vi "FPGA_main.vi"   [LabVIEW 2015]
uses:
  CONTROLS/Q_main_element.ctl
  CONTROLS/Q_FPGA_element.ctl
  GLOBAL/Global_FPGA.vi
  GLOBAL/Global_ABORT.vi
  GLOBAL/Global_MAIN.vi
  <vilib>/FPGAPlugInAG/Dynamic/niLvFpga_Reset_Dynamic.vi
  <vilib>/FPGAPlugInAG/Dynamic/niLvFpga_Close_Dynamic.vi
  <vilib>/FPGAPlugInAG/PCIe-7841R/niLvFpga_Open_PCIe-7841R.vi
  <vilib>/rvi/interface/common/dynamic/niFpgaDynamicAddResources.vi
  <vilib>/Utility/error.llb/Error Cluster From Error Code.vi
  <vilib>/rvi/errors/niLvFpgaAdjustHostInterfaceError.vi
  <vilib>/FPGAPlugInAG/Dynamic/niLvFpga_Run_Dynamic.vi
  <vilib>/FPGAPlugInAG/Dynamic/niLvFpga_Abort_Dynamic.vi
  <vilib>/rvi/interface/nirviMethod/nirviMethod.xnode
  <vilib>/rvi/interface/nirviCloseFPGA/nirviCloseFPGA.xnode
  <vilib>/rvi/interface/nirviOpenFPGA/nirviOpenFPGA.xnode
  FPGA/FPGA Bitfiles/FPGAv0_FPGATarget_FPGAlasercontrol_rVrWu38G2Ac.lvbitx
  <vilib>/rvi/interface/nirviReadWriteControl/nirviReadWriteControl.xnode
  FPGA/FPGA Bitfiles/FPGAv0_FPGATarget_FPGAmeasureQPDsi_91djMVJ3FxY.lvbitx
  FPGA/FPGA Bitfiles/FPGAv0_FPGATarget_FPGAtriggercamer_8mvrEZH3eNo.lvbitx
  FPGA/FPGA Bitfiles/FPGAv0_FPGATarget_FPGAmerFISHtrigg_IvsmFeOu1pU.lvbitx
  NiFpgaLv.dll
  <vilib>/rvi/interface/Simulation/niFpgaSimulationCallBeginRW.vi
types:
  T1 = cluster{"N laser lines":i32, "N Z positions":i32, "Laser lines":i32[], "Laser power":sgl[]}
  T2 = typedef "Q_FPGA_element.ctl" = cluster{"variant":variant, "Instruction":enum16{"FPGA_idle", "FPGA_initialize", "FPGA_error", "FPGA_security_stop", "FPGA_laser", "FPGA_start_stop_measure_QPD", "FPGA_measure_QPD", "FPGA_measure_QPD_noise", "FPGA_stop_measure_QPD", "FPGA_init_autofocus", "FPGA_init_single_scan", "FPGA_stop_single_scan", "FPGA_init_merFISH", "FPGA_measure_QPD_merFISH", "FPGA_init_scan_merFISH", "FPGA_scan_merFISH", "FPGA_close_merFISH", "FPGA_stop"}}
  T3 = typedef "Q_main_element.ctl" = cluster{"variant":variant, "Instruction":enum16{"Main_idle", "Main_initialize", "Main_initialize_TDMS", "Main_initialize_Queue", "Main_error", "Main_DAQ_initialization_results", "Main_ASI_initialization_results", "Main_Piezo_initialization_results", "Main_Valve_initialization_results", "Main_Pump_initialization_results", "Main_CAMERA_initialization_results", "Main_FPGA_initialization_results", "Main_DAQ_error", "Main_ASI_error", "Main_Piezo_error", "Main_CAMERA_error", "Main_Valve_error", "Main_Pump_error", "Main_FPGA_error", "Main_start_acquiring", "Main_not_acquiring", "Main_acquiring", "Main_stop_acquiring", "Main_change_exposure", "Main_change_z_scan_parameters", "Main_define_ROI", "Main_define_mosaic", "Main_read_kinetic_time", "Main_cooler", "Main_read_temperature", "Main_save_XY", "Main_load_XY", "Main_discard_XY", "Main_move_to_XY", "Main_measure_QPD", "Main_autofocus_calibration", "Main_autofocus_initialization", "Main_autofocus_stop", "Main_save_PID", "Main_change_H_valve_position", "Main_two_way_valve", "Main_save_movie", "Main_init_single_scan", "Main_single_scan", "Main_stop_single_scan", "Main_merFISH_illumination_parameters", "Main_merFISH_buffer_probe_list", "Main_merFISH_injections_procedure", "Main_merFISH_save_setpoint", "Main_merFISH_DAPI_parameters", "Main_merFISH_Brightfield_parameters", "Main_merFISH_save_embryo_ROI", "Main_merFISH_init", "Main_merFISH_resume", "Main_merFISH_start_autofocus", "Main_merFISH_open_close_valve_merFISH", "Main_merFISH_open_close_valve_photobleaching", "Main_merFISH_hybridization", "Main_merFISH_move_to_ROI", "Main_merFISH_wait_stabilization", "Main_merFISH_move_to_REF", "Main_merFISH_scan", "Main_merFISH_photobleaching_injection", "Main_merFISH_photobleaching", "Main_merFISH_send_email", "Main_merFISH_close", "Main_STOP"}}
  T4 = cluster{"561":sgl, "641":sgl, "405":sgl, "488":sgl}
  T5 = cluster{"N laser lines":i32, "N Z positions":i32, "Laser lines":i32[], "Laser power":sgl[], "Measure QPD":bool}
  T6 = enum16{"FPGA_idle", "FPGA_initialize", "FPGA_error", "FPGA_security_stop", "FPGA_laser", "FPGA_start_stop_measure_QPD", "FPGA_measure_QPD", "FPGA_measure_QPD_noise", "FPGA_stop_measure_QPD", "FPGA_init_autofocus", "FPGA_init_single_scan", "FPGA_stop_single_scan", "FPGA_init_merFISH", "FPGA_measure_QPD_merFISH", "FPGA_init_scan_merFISH", "FPGA_scan_merFISH", "FPGA_close_merFISH", "FPGA_stop"}
  T7 = cluster{"X":sgl, "Y":sgl, "SUM":sgl, "count":u32}
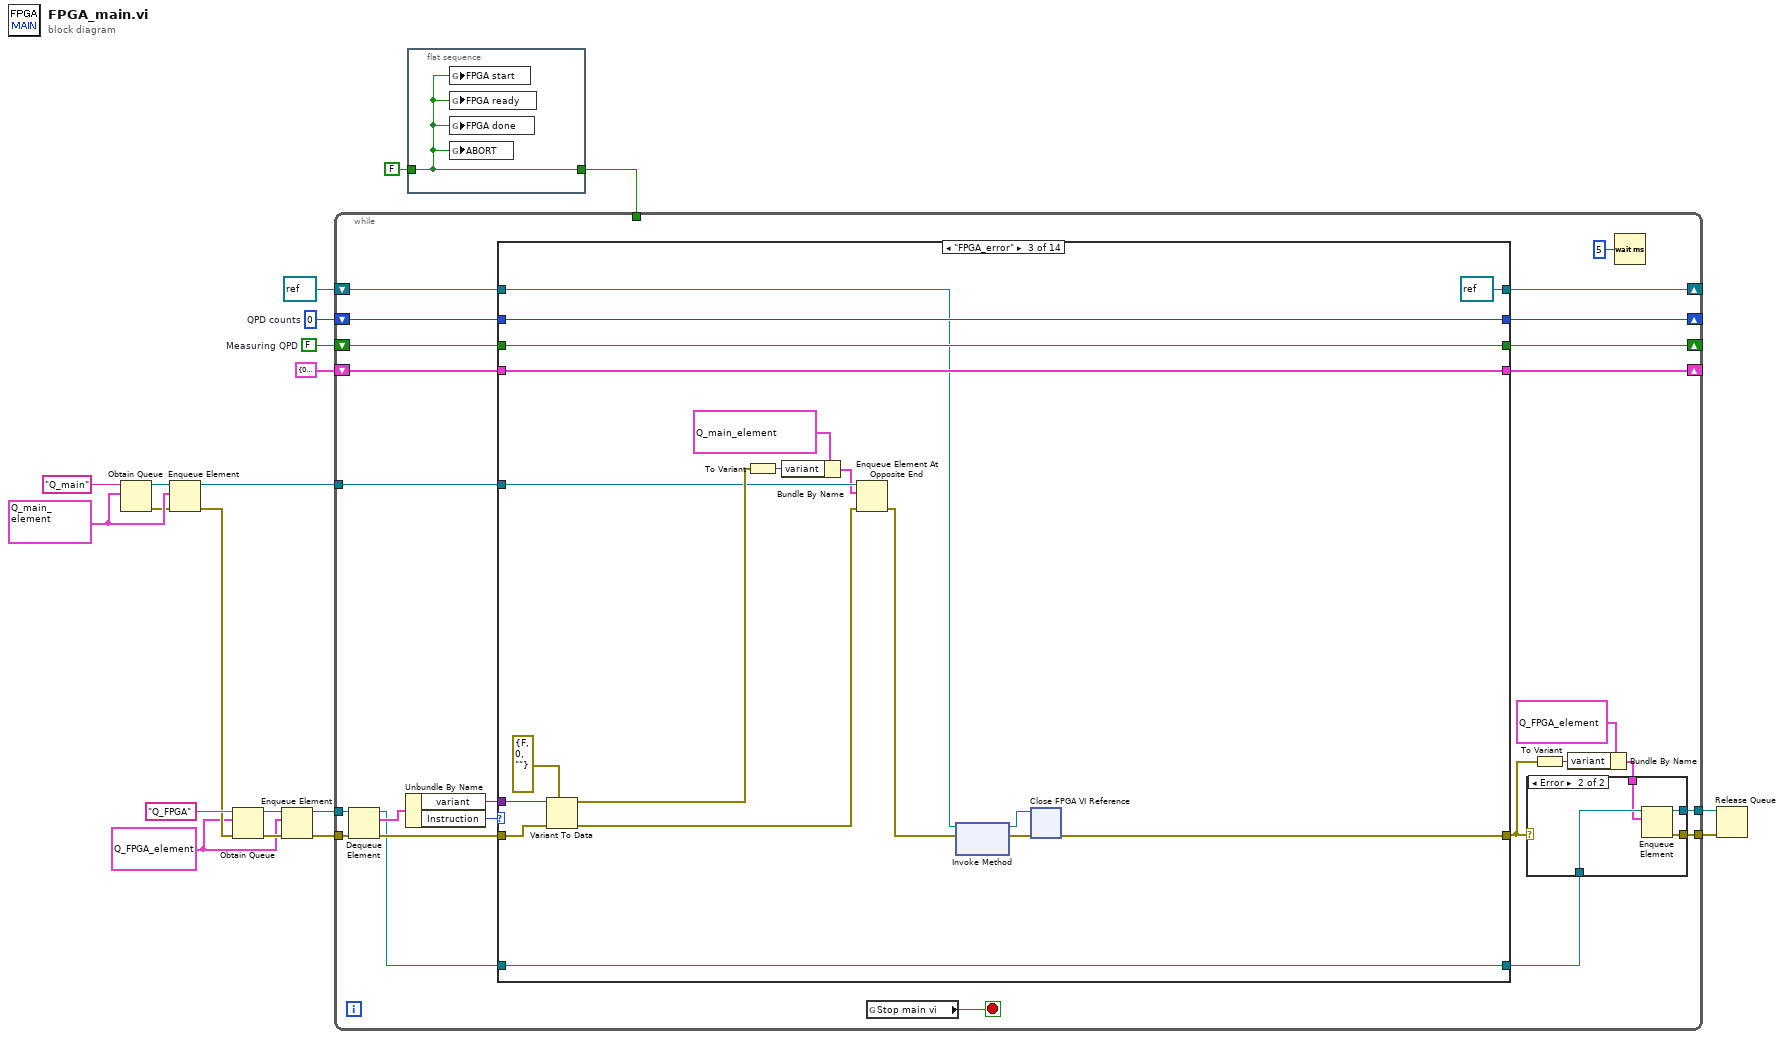
[diagram p0: block diagram]
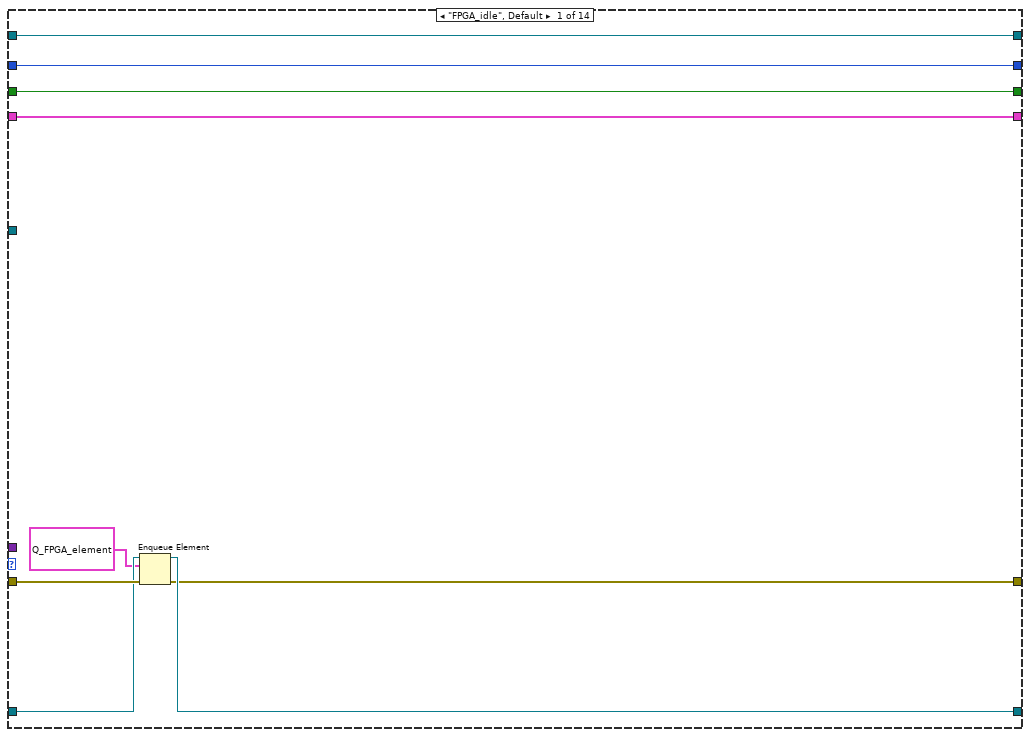
[diagram p3: hidden frame]
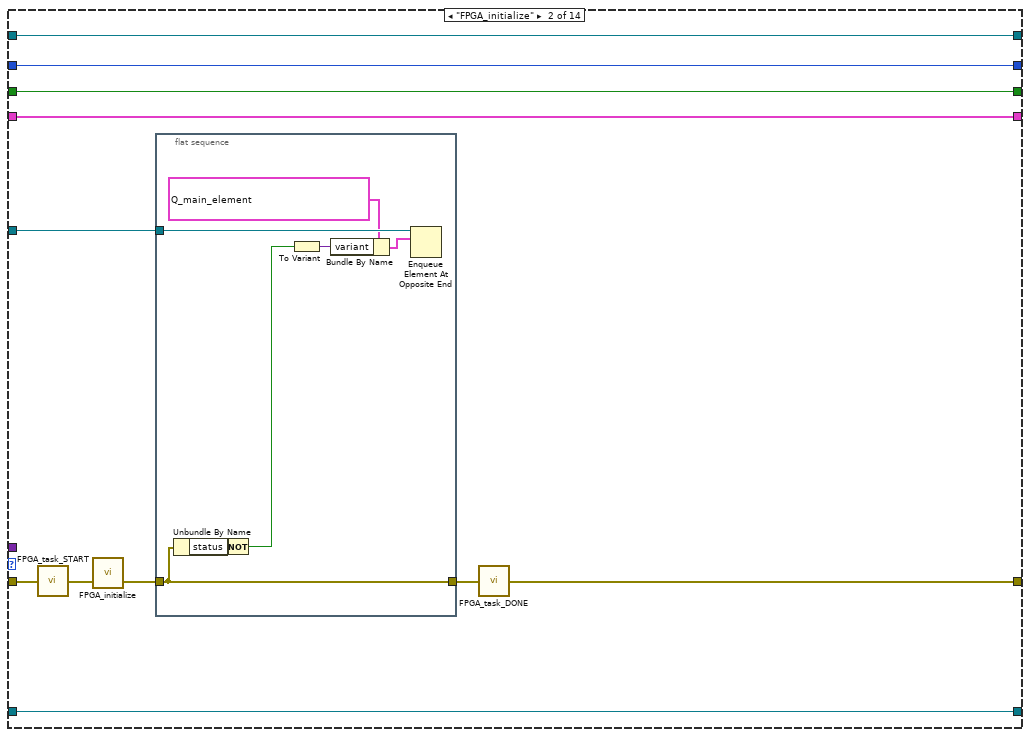
[diagram p4: hidden frame]
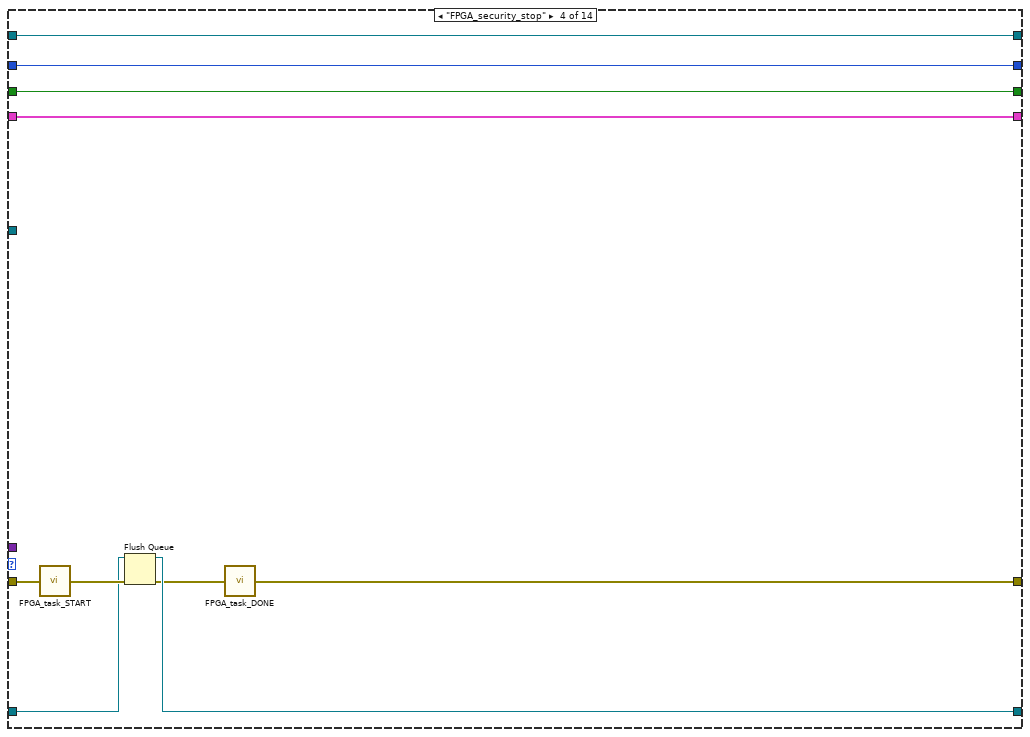
[diagram p5: hidden frame]
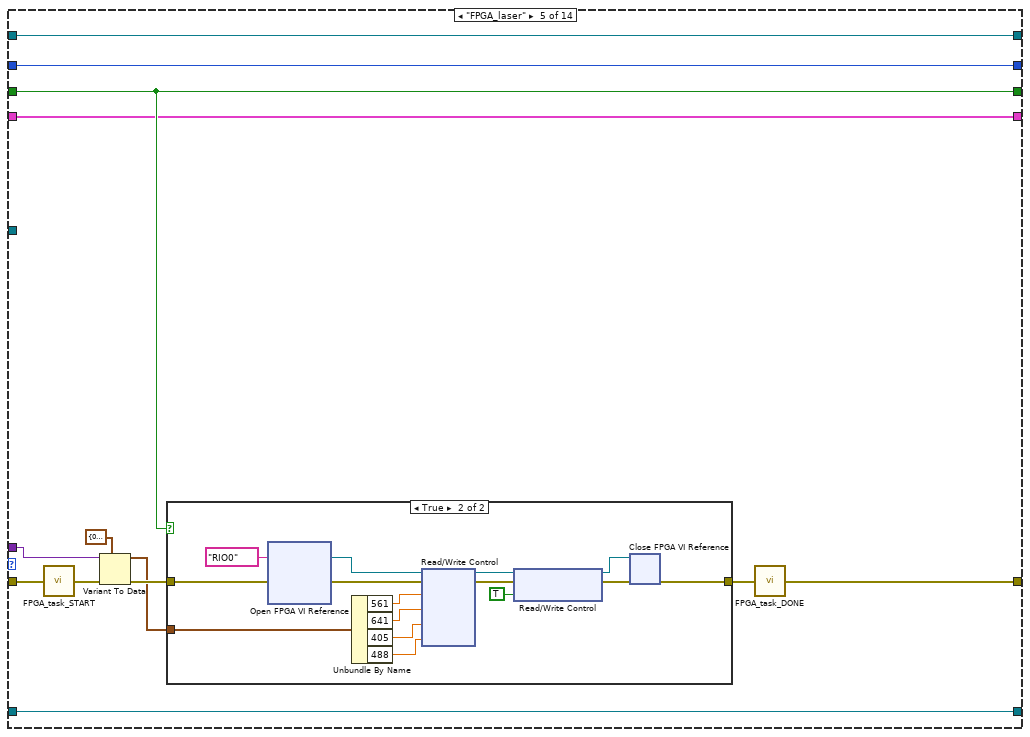
[diagram p6: hidden frame]
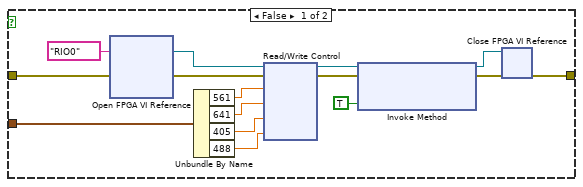
[diagram p7: hidden frame]
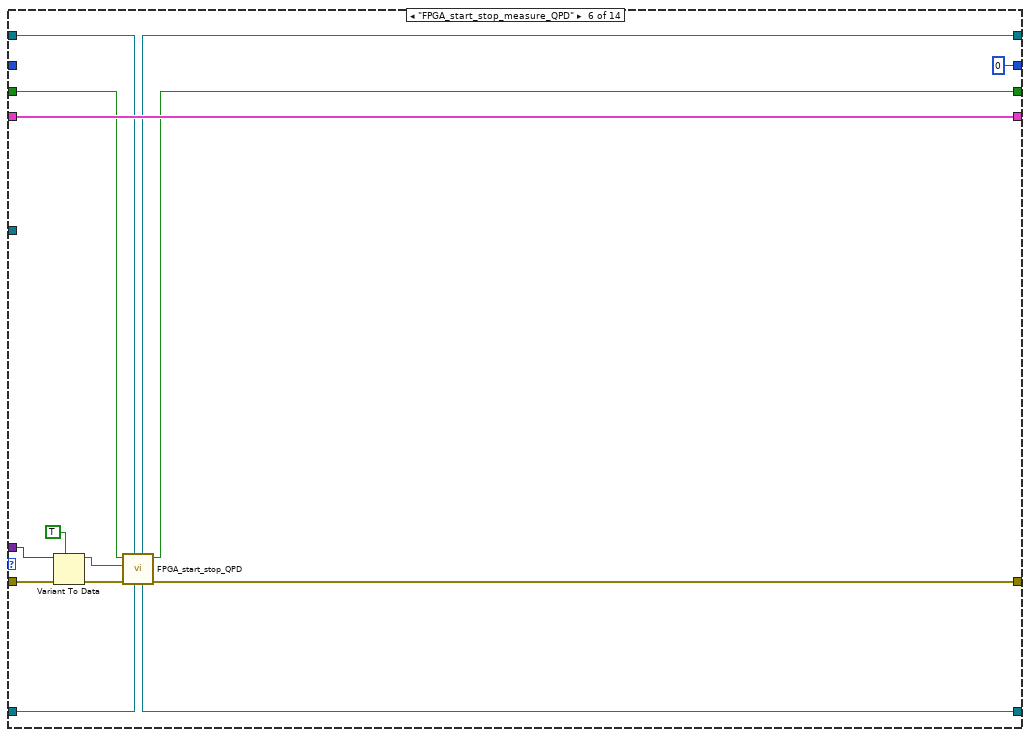
[diagram p8: hidden frame]
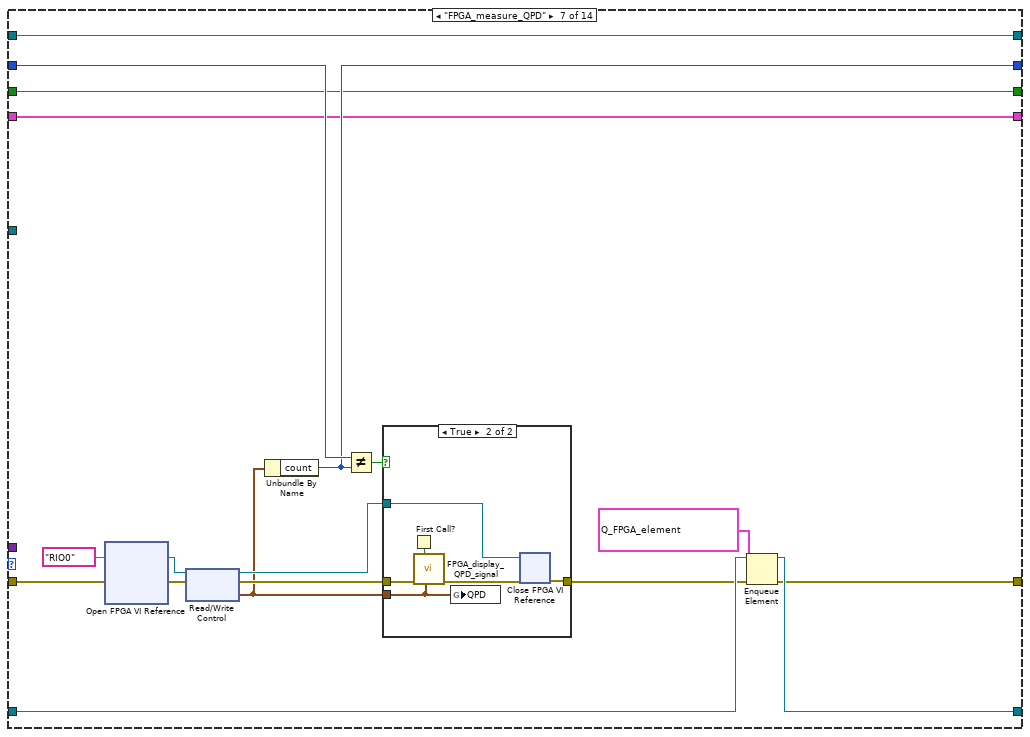
[diagram p9: hidden frame]
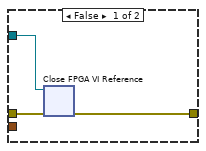
[diagram p10: hidden frame]
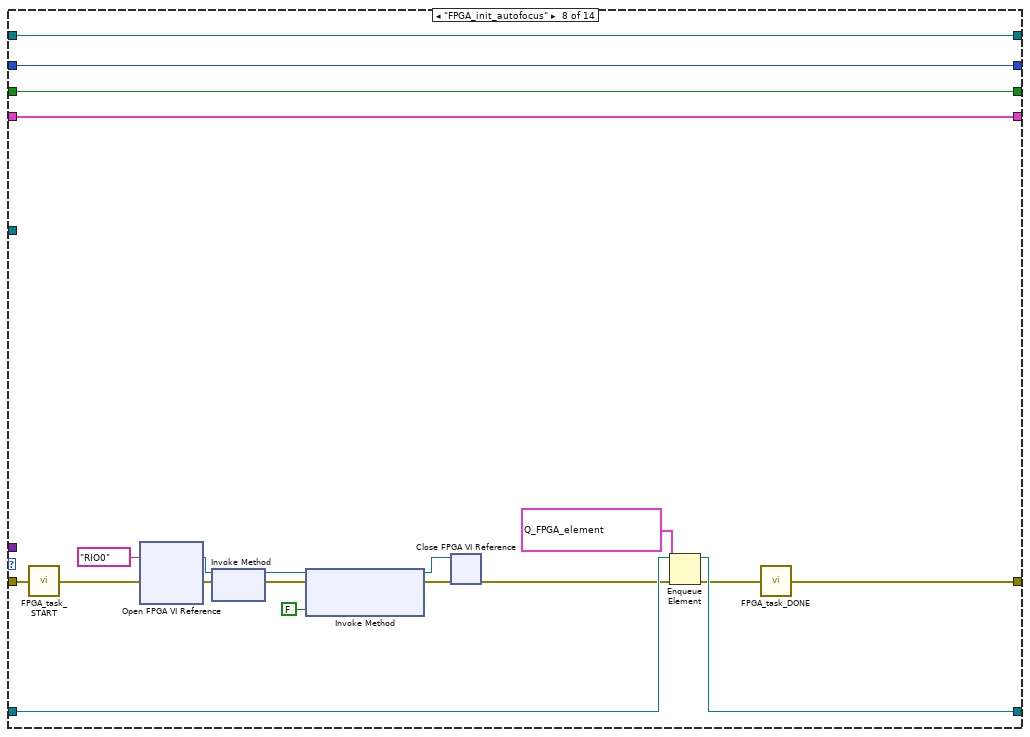
[diagram p11: hidden frame]
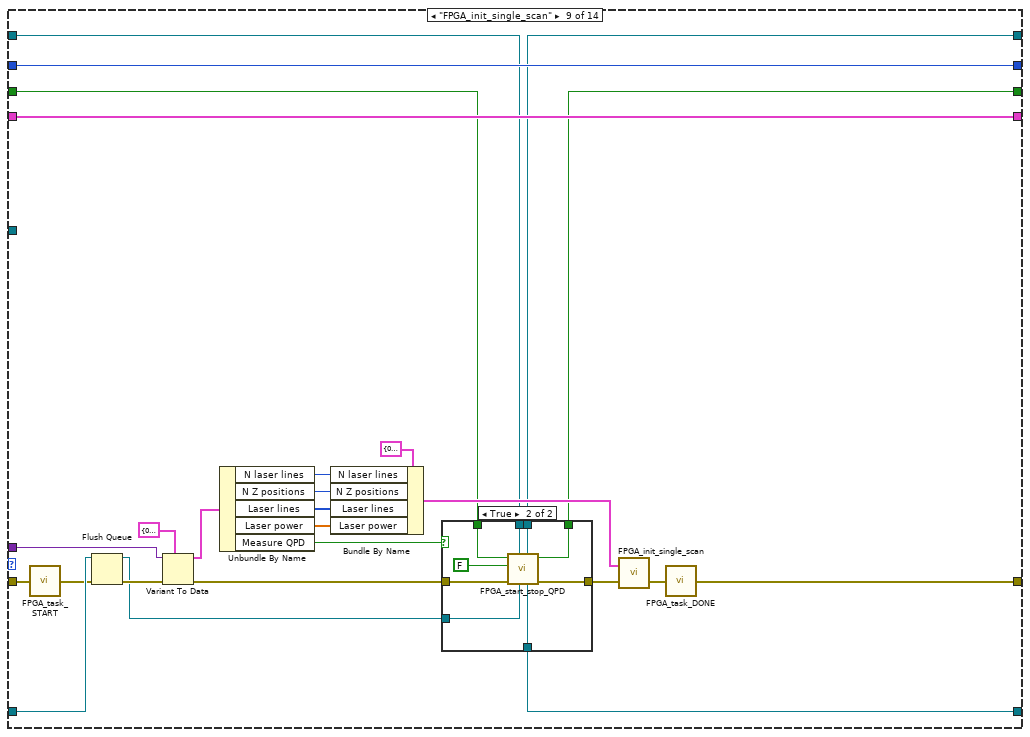
[diagram p12: hidden frame]
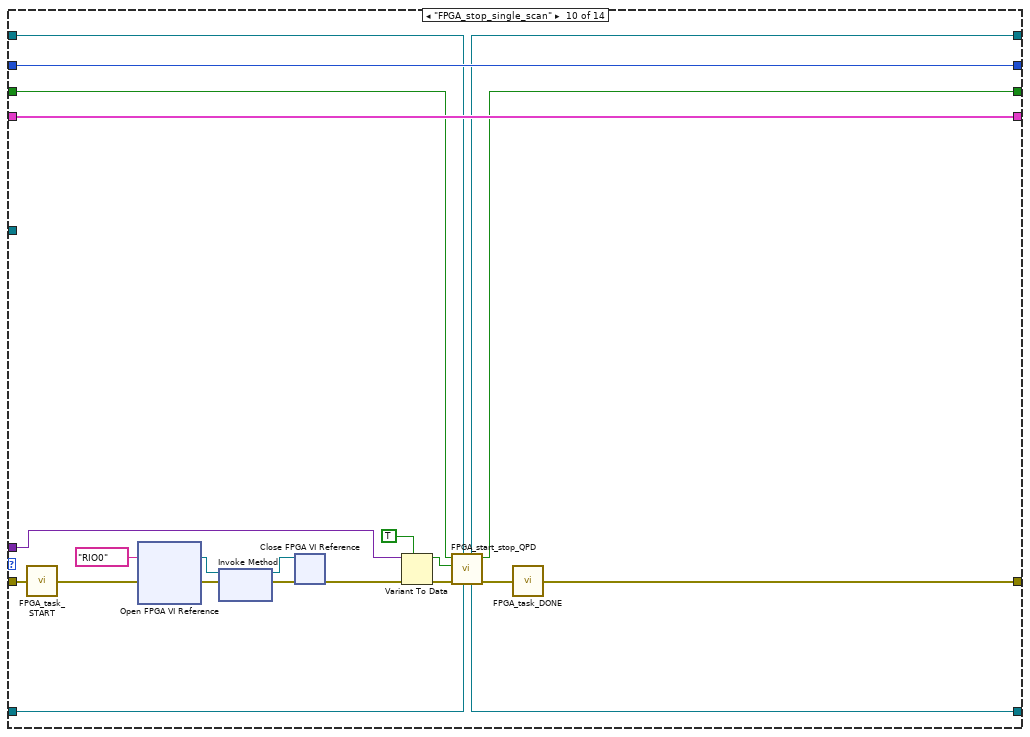
[diagram p14: hidden frame]
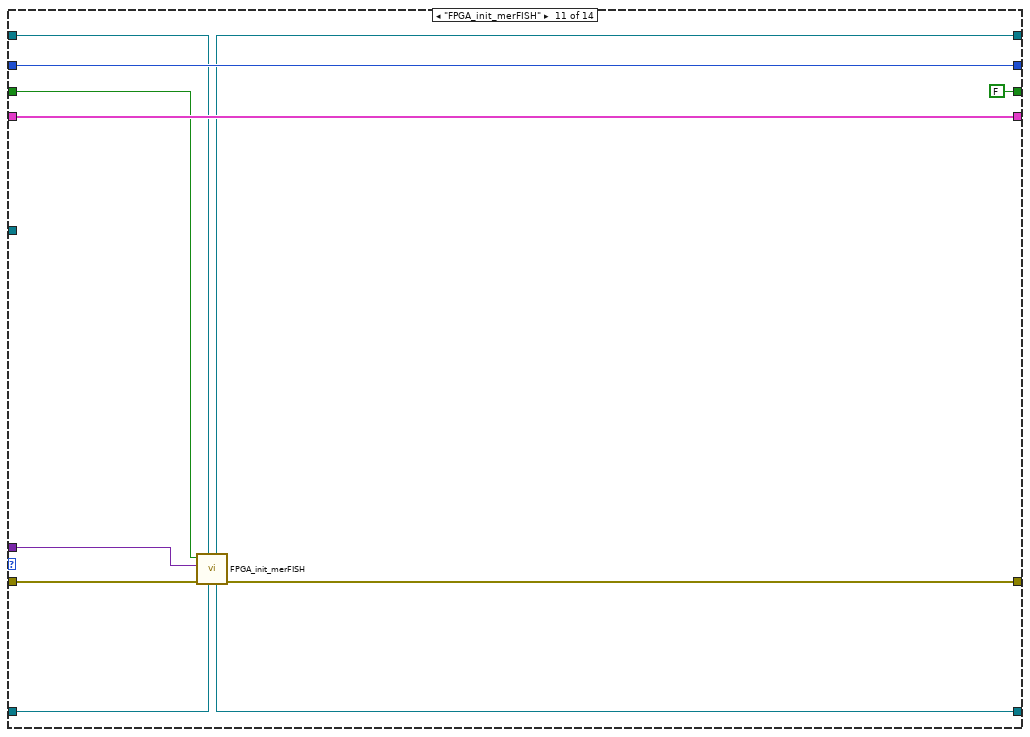
[diagram p15: hidden frame]
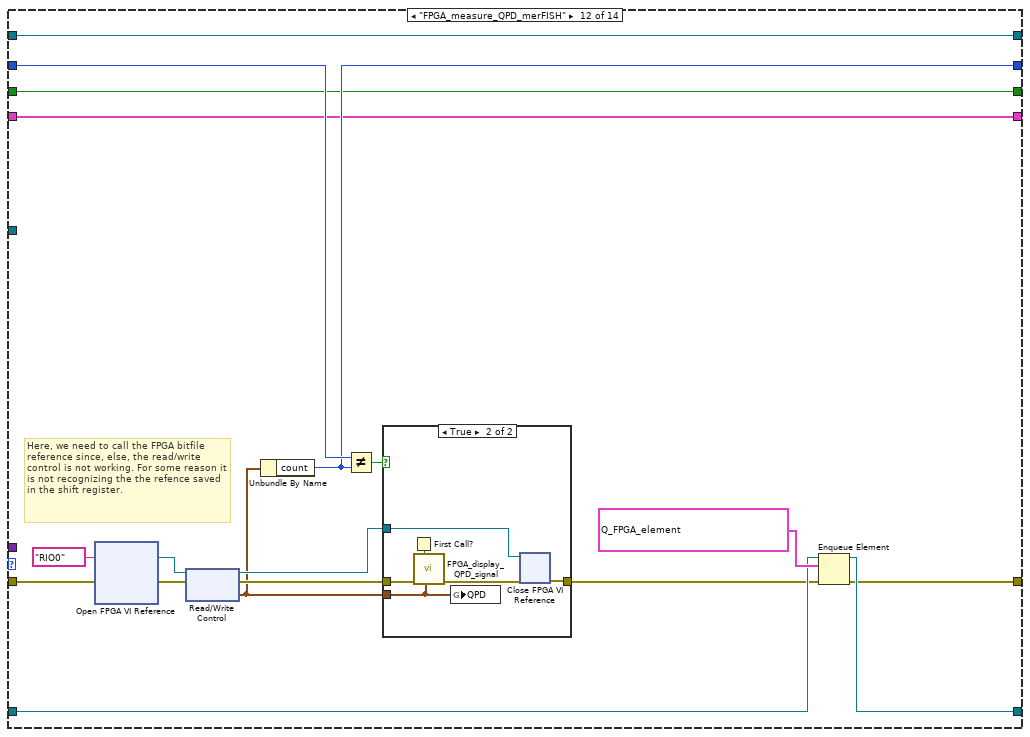
[diagram p16: hidden frame]
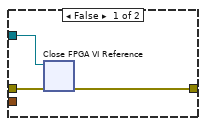
[diagram p17: hidden frame]
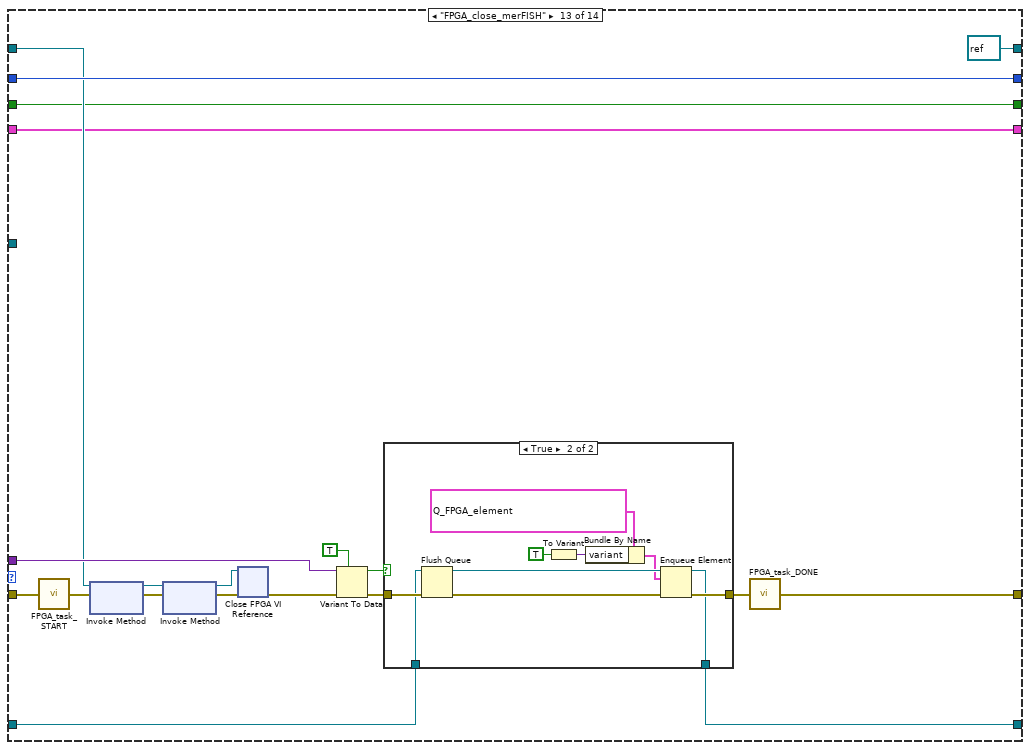
[diagram p18: hidden frame]
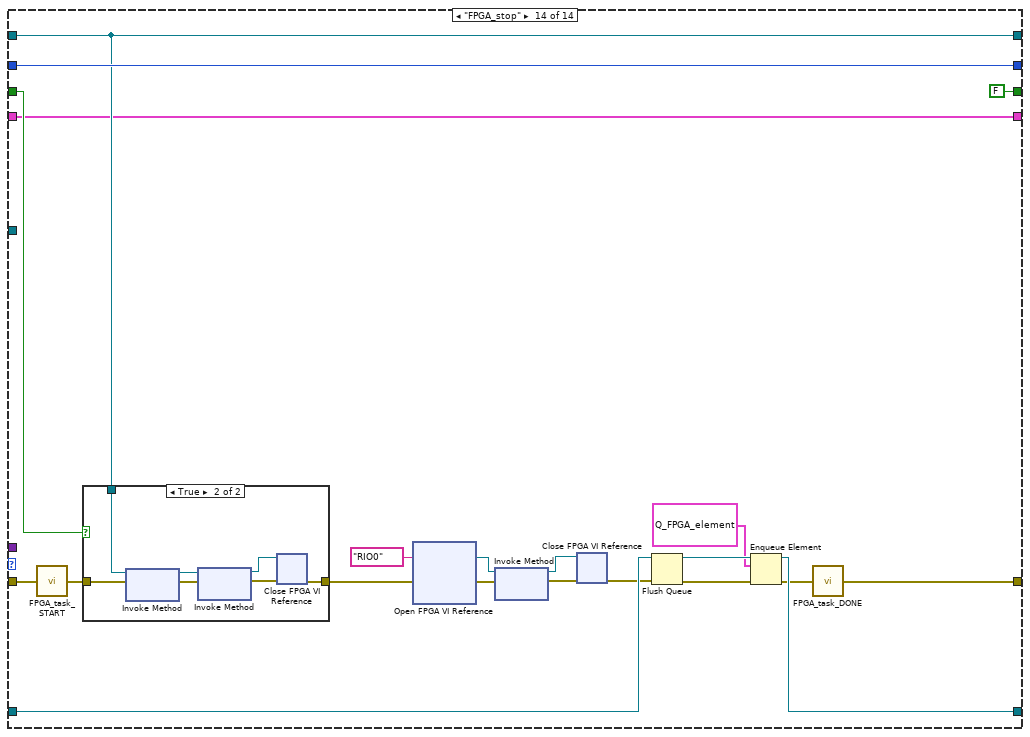
[diagram p20: hidden frame]
diagram:
  w2 = FALSE  # Measuring QPD
  w3 = u32 0  # QPD counts
  w5 = T2 {"variant"=variant, "Instruction"=enum."FPGA_idle"} ("Q_VALVE")
  w13 = T3 {"variant"=variant, "Instruction"=enum."Main_idle"} ("Q_main_element")
  n1 = Obtain Queue(name (unnamed)="Q_main", element data type=w13) -> (queue out=w11:refnum<queue>, error out=w12:errorcluster)  [unwired: 3 in, 1 out]
  n2 = Enqueue Element(queue=w11, element=w13, error in (no error)=w12) -> (queue out=w9:refnum<queue>, error out=w6:errorcluster)  [unwired: 1 in, 1 out]
  n3 = Obtain Queue(name (unnamed)="Q_FPGA", element data type=w5, error in (no error)=w6) -> (queue out=w19:refnum<queue>, error out=w18:errorcluster)  [unwired: 2 in, 1 out]
  n4 = Enqueue Element(queue=w19, element=w5, error in (no error)=w18) -> (queue out=w17:refnum<queue>, error out=w16:errorcluster)  [unwired: 1 in, 1 out]
  n5 = while {
    tunnel: w17 -> [w44]
    tunnel: w16 -> [w43]
    tunnel: [w40] -> w15
    tunnel: [w39] -> w14
    tunnel: w9 -> [w38]
    tunnel: w7 -> [_]
    shift-right: [w28] -> _
    shift-left: refnum<k20> refnum ("FPGA VI Reference Out") -> [w27]
    shift-right: [w25] -> _
    shift-left: w3 -> [w26]
    shift-right: [w23] -> _
    shift-left: w2 -> [w24]
    shift-right: [w22] -> _
    shift-left: T1 {"N laser lines"=0, "N Z positions"=0, "Laser lines"=[0, 0, 0, 0, 0], "Laser power"=[0.0, 0.0, 0.0, 0.0, 0.0]} ("FPGA cluster") -> [w21]
    stop <- w45 stop-if-true
    n6 = Dequeue Element(queue=w44, error in (no error)=w43) -> (queue out=w33:refnum<queue>, element=w42:T2, error out=w41:errorcluster)  [unwired: 1 in, 1 out]
    n7 = Unbundle By Name(w42) -> ("variant"=w37:variant, "Instruction"=w29:T6)
    n8 = case shown="\"FPGA_error\"" w29 {
      tunnel: w41 -> [w60 w69 w96 w107 w120 w155 w182 w209 w229 w272 w281 w301 w323 w358]
      tunnel: [w57 w68 w82 w104 w109 w162 w174 w207 w237 w269 w280 w293 w320 w356] -> w34
      tunnel: w38 -> [_ w71 w91 _ _ _ _ _ _ _ _ _ _ _]
      tunnel: w37 -> [_ _ w97 _ w119 w154 _ _ w236 w255 w277 _ w328 _]
      tunnel: w33 -> [w59 w70 w88 w105 w115 w161 w176 w211 w232 w262 w279 w295 w325 w363]
      tunnel: [w58 w70 w88 w103 w115 w160 w175 w210 w225 w261 w278 w294 w324 w359] -> w32
      tunnel: [w55 w67 refnum<k20> refnum ("FPGA VI Reference Out") w101 w114 w158 w171 w196 w213 w253 w273 w290 refnum<k20> refnum ("FPGA VI Reference Out") w351] -> w28
      tunnel: w27 -> [w55 w67 w80 w101 w114 w159 w171 w196 w214 w254 w274 w290 w318 w351]
      tunnel: w26 -> [w54 w66 w87 w100 w111 _ w169 w202 w235 w268 w283 w288 w319 w355]
      tunnel: [w54 w66 w87 w100 w111 u32 0 ("QPD counts") w167 w202 w235 w268 w283 w286 w319 w355] -> w25
      tunnel: w24 -> [w53 w65 w81 w99 w110 w157 w166 w201 w216 w252 w276 w285 w317 w353]
      tunnel: [w53 w65 w81 w99 w110 w151 w166 w201 w215 w251 FALSE ("Measuring QPD") w285 w317 FALSE ("Measuring QPD")] -> w23
      tunnel: [w52 w64 w86 w98 w108 w163 w165 w192 w234 w264 w282 w284 w315 w350] -> w22
      tunnel: w21 -> [w52 w64 w86 w98 w108 w163 w165 w192 w234 w264 w282 w284 w315 w350]
      frame "FPGA_idle", Default {
        n9 = Enqueue Element(queue=w59, element=T2 {"variant"=variant, "Instruction"=enum."FPGA_idle"} ("Q_VALVE"), error in (no error)=w60) -> (queue out=w58:refnum<queue>, error out=w57:errorcluster)  [unwired: 1 in, 1 out]
      }
      frame "FPGA_initialize" {
        n10 = call "FPGA_task_START.vi"("error in"=w69) -> ("error out"=w63:errorcluster)
        n11 = call "FPGA_initialize.vi"("error in"=w63) -> ("error out"=w62:errorcluster)  [unwired: 2 in]
        n12 = flat-sequence {
          tunnel: w71 -> [w78]
          tunnel: w62 -> [w74]
          tunnel: [w74] -> w61
          frame #0 {
            n13 = Unbundle By Name(w74) -> ("status"=w73:bool)
            n14 = Not(x=w73) -> (.not. x?=w72:bool)
            n15 = To Variant(anything=w72) -> (Variant=w76:variant)
            n16 = Bundle By Name(cluster=T3 {"variant"=variant, "Instruction"=enum."Main_FPGA_initialization_results"} ("element"), "variant"=w76) -> (w75:T3)
            n17 = Enqueue Element At Opposite End(queue=w78, element=w75) -> ()  [unwired: 2 in, 3 out]
          }
        }
        n18 = call "FPGA_task_DONE.vi"("error in"=w61) -> ("error out"=w68:errorcluster)
      }
      frame "FPGA_error" {
        n19 = Variant To Data(error in=w96, type=errorcluster {"status"=FALSE, "code"=0, "source"=""} ("error out"), Variant=w97) -> (data=w92:errorcluster, error out=w90:errorcluster)
        n20 = To Variant(anything=w92) -> (Variant=w93:variant)
        n21 = Bundle By Name(cluster=T3 {"variant"=variant, "Instruction"=enum."Main_FPGA_error"} ("Q_main_element"), "variant"=w93) -> (w89:T3)
        n22 = Enqueue Element At Opposite End(queue=w91, element=w89, error in (no error)=w90) -> (error out=w83:errorcluster)  [unwired: 1 in, 2 out]
        n23 = xnode "Invoke Method"("FPGA VI Reference In"=w80, "error in"=w83) -> ("FPGA VI Reference Out"=w85:refnum<k20>, "error out"=w84:errorcluster)
        n24 = xnode "Close FPGA VI Reference"("FPGA VI Reference In"=w85, "error in"=w84) -> ("error out"=w82:errorcluster)
      }
      frame "FPGA_security_stop" {
        n25 = call "FPGA_task_START.vi"("error in"=w107) -> ("error out"=w106:errorcluster)
        n26 = Flush Queue(queue=w105, error in (no error)=w106) -> (queue out=w103:refnum<queue>, error out=w102:errorcluster)  [unwired: 1 out]
        n27 = call "FPGA_task_DONE.vi"("error in"=w102) -> ("error out"=w104:errorcluster)
      }
      frame "FPGA_laser" {
        n28 = call "FPGA_task_START.vi"("error in"=w120) -> ("error out"=w113:errorcluster)
        n29 = Variant To Data(error in=w113, type=T4 {"561"=0.0, "641"=0.0, "405"=0.0, "488"=0.0} ("output cluster"), Variant=w119) -> (data=w117:T4, error out=w118:errorcluster)
        n30 = case shown="True" w110 {
          tunnel: w118 -> [w132 w147]
          tunnel: w117 -> [w131 w146]
          tunnel: [w122 w142] -> w116
          frame False {
            n31 = xnode "Open FPGA VI Reference"("error in"=w132, "resource name"=tag "RIO0") -> ("FPGA VI Reference Out"=w133:refnum<k20>, "error out"=w134:errorcluster)
            n32 = Unbundle By Name(w131) -> ("561"=w130:sgl, "641"=w129:sgl, "405"=w121:sgl, "488"=w128:sgl)
            n33 = xnode "Read/Write Control"("FPGA VI Reference In"=w133, "error in"=w134, "561"=w130, "640"=w129, "405"=w121, "488"=w128) -> ("FPGA VI Reference Out"=w127:refnum<k20>, "error out"=w126:errorcluster)
            n34 = xnode "Invoke Method"("FPGA VI Reference In"=w127, "error in"=w126, "Wait Until Done (F)"=TRUE) -> ("FPGA VI Reference Out"=w123:refnum<k20>, "error out"=w124:errorcluster)
            n35 = xnode "Close FPGA VI Reference"("FPGA VI Reference In"=w123, "error in"=w124) -> ("error out"=w122:errorcluster)
          }
          frame True {
            n36 = xnode "Open FPGA VI Reference"("error in"=w147, "resource name"=tag "RIO0") -> ("FPGA VI Reference Out"=w148:refnum<k20>, "error out"=w149:errorcluster)
            n37 = Unbundle By Name(w146) -> ("561"=w145:sgl, "641"=w144:sgl, "405"=w141:sgl, "488"=w143:sgl)
            n38 = xnode "Read/Write Control"("FPGA VI Reference In"=w148, "error in"=w149, "561"=w145, "640"=w144, "405"=w141, "488"=w143) -> ("FPGA VI Reference Out"=w140:refnum<k20>, "error out"=w139:errorcluster)
            n39 = xnode "Read/Write Control"("FPGA VI Reference In"=w140, "error in"=w139, "Update lasers"=TRUE) -> ("FPGA VI Reference Out"=w136:refnum<k20>, "error out"=w137:errorcluster)
            n40 = xnode "Close FPGA VI Reference"("FPGA VI Reference In"=w136, "error in"=w137) -> ("error out"=w142:errorcluster)
          }
        }
        n41 = call "FPGA_task_DONE.vi"("error in"=w116) -> ("error out"=w109:errorcluster)
      }
      frame "FPGA_start_stop_measure_QPD" {
        n42 = Variant To Data(error in=w155, type=TRUE, Variant=w154) -> (data=w153:bool, error out=w152:errorcluster)
        n43 = call "FPGA_start_stop_QPD.vi"("queue FPGA IN"=w161, "FPGA VI Reference IN"=w159, "error in"=w152, "start ?"=w153, "Measuring QPD"=w157) -> ("error out"=w162:errorcluster, "Measuring QPD"=w151:bool, "queue FPGA OUT"=w160:refnum<queue>, "FPGA VI Reference OUT"=w158:refnum<k20>)  [unwired: 3 in]
      }
      frame "FPGA_measure_QPD" {
        n44 = xnode "Open FPGA VI Reference"("error in"=w182, "resource name"=tag "RIO0") -> ("FPGA VI Reference Out"=w179:refnum<k20>, "error out"=w180:errorcluster)
        n45 = xnode "Read/Write Control"("FPGA VI Reference In"=w179, "error in"=w180) -> ("FPGA VI Reference Out"=w172:refnum<k20>, "error out"=w178:errorcluster, "QPD"=w170:T7)
        n46 = Unbundle By Name(w170) -> ("count"=w167:u32)
        n47 = Not Equal?(x=w169, y=w167) -> (x != y?=w168:bool)
        n48 = case shown="True" w168 {
          tunnel: w178 -> [w185 w189]
          tunnel: [w183 w188] -> w173
          tunnel: w170 -> [_ w190]
          tunnel: w172 -> [w184 w186]
          frame False {
            n49 = xnode "Close FPGA VI Reference"("FPGA VI Reference In"=w184, "error in"=w185) -> ("error out"=w183:errorcluster)
          }
          frame True {
            n50 = First Call?() -> (First Call?: T/F=w191:bool)
            n51 = call "FPGA_display_QPD_signal.vi"("QPD"=w190, "Reset"=w191, "error in"=w189) -> ("error out"=w187:errorcluster)  [unwired: 6 in]
            n52 = global write "Global_FPGA.vi" "QPD"(w190) -> ()
            n53 = xnode "Close FPGA VI Reference"("FPGA VI Reference In"=w186, "error in"=w187) -> ("error out"=w188:errorcluster)
          }
        }
        n54 = Enqueue Element(queue=w176, element=T2 {"variant"=variant, "Instruction"=enum."FPGA_measure_QPD"}, error in (no error)=w173) -> (queue out=w175:refnum<queue>, error out=w174:errorcluster)  [unwired: 1 in, 1 out]
      }
      frame "FPGA_init_autofocus" {
        n55 = call "FPGA_task_START.vi"("error in"=w209) -> ("error out"=w200:errorcluster)
        n56 = xnode "Open FPGA VI Reference"("error in"=w200, "resource name"=tag "RIO0") -> ("FPGA VI Reference Out"=w198:refnum<k20>, "error out"=w199:errorcluster)
        n57 = xnode "Invoke Method"("FPGA VI Reference In"=w198, "error in"=w199) -> ("FPGA VI Reference Out"=w205:refnum<k20>, "error out"=w204:errorcluster)
        n58 = xnode "Invoke Method"("FPGA VI Reference In"=w205, "error in"=w204, "Wait Until Done (F)"=FALSE) -> ("FPGA VI Reference Out"=w194:refnum<k20>, "error out"=w195:errorcluster)
        n59 = xnode "Close FPGA VI Reference"("FPGA VI Reference In"=w194, "error in"=w195) -> ("error out"=w193:errorcluster)
        n60 = Enqueue Element(queue=w211, element=T2 {"variant"=variant, "Instruction"=enum."FPGA_measure_QPD"}, error in (no error)=w193) -> (queue out=w210:refnum<queue>, error out=w208:errorcluster)  [unwired: 1 in, 1 out]
        n61 = call "FPGA_task_DONE.vi"("error in"=w208) -> ("error out"=w207:errorcluster)
      }
      frame "FPGA_init_single_scan" {
        n62 = call "FPGA_task_START.vi"("error in"=w229) -> ("error out"=w228:errorcluster)
        n63 = Flush Queue(queue=w232, error in (no error)=w228) -> (queue out=w226:refnum<queue>, error out=w231:errorcluster)  [unwired: 1 out]
        n64 = Variant To Data(error in=w231, type=T5 {"N laser lines"=0, "N Z positions"=0, "Laser lines"=[0, 0, 0, 0, 0], "Laser power"=[0.0, 0.0, 0.0, 0.0, 0.0], "Measure QPD"=FALSE} ("output cluster"), Variant=w236) -> (data=w223:T5, error out=w227:errorcluster)
        n65 = Unbundle By Name(w223) -> ("N laser lines"=w221:i32, "N Z positions"=w220:i32, "Laser lines"=w219:i32[], "Laser power"=w218:sgl[], "Measure QPD"=w212:bool)
        n66 = Bundle By Name(cluster=T1 {"N laser lines"=0, "N Z positions"=0, "Laser lines"=[], "Laser power"=[]} ("data"), "N laser lines"=w221, "N Z positions"=w220, "Laser lines"=w219, "Laser power"=w218) -> (w217:T1)
        n67 = case shown="True" w212 {
          tunnel: w227 -> [w238 w250]
          tunnel: w226 -> [w239 w249]
          tunnel: [w239 w248] -> w225
          tunnel: [w238 w247] -> w224
          tunnel: w216 -> [w240 w246]
          tunnel: [w240 w245] -> w215
          tunnel: w214 -> [w241 w244]
          tunnel: [w241 w243] -> w213
          frame False {
          }
          frame True {
            n68 = call "FPGA_start_stop_QPD.vi"("queue FPGA IN"=w249, "FPGA VI Reference IN"=w244, "error in"=w250, "start ?"=FALSE, "Measuring QPD"=w246) -> ("error out"=w247:errorcluster, "Measuring QPD"=w245:bool, "queue FPGA OUT"=w248:refnum<queue>, "FPGA VI Reference OUT"=w243:refnum<k20>)  [unwired: 3 in]
          }
        }
        n69 = call "FPGA_init_single_scan.vi"("error in"=w224, "data"=w217) -> ("error out"=w233:errorcluster)  [unwired: 1 in]
        n70 = call "FPGA_task_DONE.vi"("error in"=w233) -> ("error out"=w237:errorcluster)
      }
      frame "FPGA_stop_single_scan" {
        n71 = call "FPGA_task_START.vi"("error in"=w272) -> ("error out"=w259:errorcluster)
        n72 = xnode "Open FPGA VI Reference"("error in"=w259, "resource name"=tag "RIO0") -> ("FPGA VI Reference Out"=w265:refnum<k20>, "error out"=w266:errorcluster)
        n73 = xnode "Invoke Method"("FPGA VI Reference In"=w265, "error in"=w266) -> ("FPGA VI Reference Out"=w270:refnum<k20>, "error out"=w271:errorcluster)
        n74 = xnode "Close FPGA VI Reference"("FPGA VI Reference In"=w270, "error in"=w271) -> ("error out"=w258:errorcluster)
        n75 = Variant To Data(error in=w258, type=TRUE, Variant=w255) -> (data=w256:bool, error out=w257:errorcluster)
        n76 = call "FPGA_start_stop_QPD.vi"("queue FPGA IN"=w262, "FPGA VI Reference IN"=w254, "error in"=w257, "start ?"=w256, "Measuring QPD"=w252) -> ("error out"=w263:errorcluster, "Measuring QPD"=w251:bool, "queue FPGA OUT"=w261:refnum<queue>, "FPGA VI Reference OUT"=w253:refnum<k20>)  [unwired: 3 in]
        n77 = call "FPGA_task_DONE.vi"("error in"=w263) -> ("error out"=w269:errorcluster)
      }
      frame "FPGA_init_merFISH" {
        n78 = call "FPGA_init_merFISH.vi"("queue FPGA IN"=w279, "FPGA VI Reference in"=w274, "error in"=w281, "variant"=w277, "Measuring QPD"=w276) -> ("error out"=w280:errorcluster, "queue FPGA OUT"=w278:refnum<queue>, "FPGA VI Reference Out"=w273:refnum<k20>)  [unwired: 4 in]
      }
      frame "FPGA_measure_QPD_merFISH" {
        # "Here, we need to call the FPGA bitfile reference since, else, the read/write control is not working. For some reason it is not recognizing the the refence saved in the shift register."
        n79 = xnode "Open FPGA VI Reference"("error in"=w301, "resource name"=tag "RIO0") -> ("FPGA VI Reference Out"=w298:refnum<k20>, "error out"=w299:errorcluster)
        n80 = xnode "Read/Write Control"("FPGA VI Reference In"=w298, "error in"=w299) -> ("FPGA VI Reference Out"=w291:refnum<k20>, "error out"=w297:errorcluster, "QPD"=w289:T7)
        n81 = Unbundle By Name(w289) -> ("count"=w286:u32)
        n82 = Not Equal?(x=w288, y=w286) -> (x != y?=w287:bool)
        n83 = case shown="True" w287 {
          tunnel: w297 -> [w304 w308]
          tunnel: [w302 w307] -> w292
          tunnel: w289 -> [_ w309]
          tunnel: w291 -> [w303 w305]
          frame False {
            n84 = xnode "Close FPGA VI Reference"("FPGA VI Reference In"=w303, "error in"=w304) -> ("error out"=w302:errorcluster)
          }
          frame True {
            n85 = First Call?() -> (First Call?: T/F=w310:bool)
            n86 = call "FPGA_display_QPD_signal.vi"("QPD"=w309, "Reset"=w310, "error in"=w308) -> ("error out"=w306:errorcluster)  [unwired: 6 in]
            n87 = global write "Global_FPGA.vi" "QPD"(w309) -> ()
            n88 = xnode "Close FPGA VI Reference"("FPGA VI Reference In"=w305, "error in"=w306) -> ("error out"=w307:errorcluster)
          }
        }
        n89 = Enqueue Element(queue=w295, element=T2 {"variant"=variant, "Instruction"=enum."FPGA_measure_QPD_merFISH"}, error in (no error)=w292) -> (queue out=w294:refnum<queue>, error out=w293:errorcluster)  [unwired: 1 in, 1 out]
      }
      frame "FPGA_close_merFISH" {
        n90 = call "FPGA_task_START.vi"("error in"=w323) -> ("error out"=w322:errorcluster)
        n91 = xnode "Invoke Method"("FPGA VI Reference In"=w318, "error in"=w322) -> ("FPGA VI Reference Out"=w314:refnum<k20>, "error out"=w313:errorcluster)
        n92 = xnode "Invoke Method"("FPGA VI Reference In"=w314, "error in"=w313) -> ("FPGA VI Reference Out"=w311:refnum<k20>, "error out"=w312:errorcluster)
        n93 = xnode "Close FPGA VI Reference"("FPGA VI Reference In"=w311, "error in"=w312) -> ("error out"=w330:errorcluster)
        n94 = Variant To Data(error in=w330, type=TRUE, Variant=w328) -> (data=w327:bool, error out=w326:errorcluster)
        n95 = case shown="True" w327 {
          tunnel: w326 -> [w331 w338]
          tunnel: w325 -> [w332 w337]
          tunnel: [w331 w334] -> w321
          tunnel: [w332 w333] -> w324
          frame False {
          }
          frame True {
            n96 = Flush Queue(queue=w337, error in (no error)=w338) -> (queue out=w340:refnum<queue>, error out=w339:errorcluster)  [unwired: 1 out]
            n97 = To Variant(anything=TRUE) -> (Variant=w342:variant)
            n98 = Bundle By Name(cluster=T2 {"variant"=variant, "Instruction"=enum."FPGA_start_stop_measure_QPD"} ("element"), "variant"=w342) -> (w335:T2)
            n99 = Enqueue Element(queue=w340, element=w335, error in (no error)=w339) -> (queue out=w333:refnum<queue>, error out=w334:errorcluster)  [unwired: 1 in, 1 out]
          }
        }
        n100 = call "FPGA_task_DONE.vi"("error in"=w321) -> ("error out"=w320:errorcluster)
      }
      frame "FPGA_stop" {
        n101 = call "FPGA_task_START.vi"("error in"=w358) -> ("error out"=w354:errorcluster)
        n102 = case shown="True" w353 {
          tunnel: w354 -> [w364 w365]
          tunnel: [w364 w371] -> w348
          tunnel: w351 -> [_ w366]
          frame False {
          }
          frame True {
            n103 = xnode "Invoke Method"("FPGA VI Reference In"=w366, "error in"=w365) -> ("FPGA VI Reference Out"=w370:refnum<k20>, "error out"=w369:errorcluster)
            n104 = xnode "Invoke Method"("FPGA VI Reference In"=w370, "error in"=w369) -> ("FPGA VI Reference Out"=w367:refnum<k20>, "error out"=w368:errorcluster)
            n105 = xnode "Close FPGA VI Reference"("FPGA VI Reference In"=w367, "error in"=w368) -> ("error out"=w371:errorcluster)
          }
        }
        n106 = xnode "Open FPGA VI Reference"("error in"=w348, "resource name"=tag "RIO0") -> ("FPGA VI Reference Out"=w346:refnum<k20>, "error out"=w347:errorcluster)
        n107 = xnode "Invoke Method"("FPGA VI Reference In"=w346, "error in"=w347) -> ("FPGA VI Reference Out"=w344:refnum<k20>, "error out"=w345:errorcluster)
        n108 = xnode "Close FPGA VI Reference"("FPGA VI Reference In"=w344, "error in"=w345) -> ("error out"=w343:errorcluster)
        n109 = Flush Queue(queue=w363, error in (no error)=w343) -> (queue out=w361:refnum<queue>, error out=w362:errorcluster)  [unwired: 1 out]
        n110 = Enqueue Element(queue=w361, element=T2 {"variant"=variant, "Instruction"=enum."FPGA_idle"}, error in (no error)=w362) -> (queue out=w359:refnum<queue>, error out=w357:errorcluster)  [unwired: 1 in, 1 out]
        n111 = call "FPGA_task_DONE.vi"("error in"=w357) -> ("error out"=w356:errorcluster)
      }
    }
    n112 = global read "Global_MAIN.vi" "Stop main vi"() -> (w45:bool)
    n113 = To Variant(anything=w34) -> (Variant=w35:variant)
    n114 = Bundle By Name(cluster=T2 {"variant"=variant, "Instruction"=enum."FPGA_error"} ("Q_VALVE"), "variant"=w35) -> (w36:T2)
    n115 = case shown="Error" w34 {
      selector: w34 -> [w47 _]
      tunnel: [w46 w50] -> w40
      tunnel: [w47 w51] -> w39
      tunnel: w32 -> [w46 w49]
      tunnel: w36 -> [_ w48]
      frame No Error {
      }
      frame Error {
        n116 = Enqueue Element(queue=w49, element=w48) -> (queue out=w50:refnum<queue>, error out=w51:errorcluster)  [unwired: 2 in, 1 out]
      }
    }
    n117 = Wait (ms)(milliseconds to wait=u32 5) -> ()  [unwired: 1 out]
  }
  n118 = flat-sequence {
    tunnel: FALSE ("Stop main vi") -> [w372]
    tunnel: [w372] -> w7
    frame #0 {
      n119 = global write "Global_FPGA.vi" "FPGA start"(w372) -> ()
      n120 = global write "Global_FPGA.vi" "FPGA ready"(w372) -> ()
      n121 = global write "Global_FPGA.vi" "FPGA done"(w372) -> ()
      n122 = global write "Global_ABORT.vi" "ABORT"(w372) -> ()
    }
  }
  n123 = Release Queue(queue=w15, error in (no error)=w14) -> ()  [unwired: 1 in, 3 out]
